vi "find_handle_pose_update.vi"(8 "Manipulator pose":T7 format="%#_5f", 9 "Light 3":sgl[](array[numeric]), 10 "Parameters":T1={"Stimulus"={"Type"=enum."Off", "Delay"=0, "Amplitude"=[0.0, 0.0, 0.0], "Injection point"=enum."Total pose", "Closed loop"=FALSE, "Offset"=[0.0, 0.0, 0.0], "Tip -> world"=TRUE}, "Goal Filter A"={"Lower Fc"=0.0, "Lower Q"=0.15, "Scale factor"=0.0, "Upper Fc"=0.0075, "Upper Q"=0.01, "Manip zeroing"=0.001, "Speedup max"=150.0, "Speedup thresh"=5.0, "Speedup nonlin"=3.0, "V limit"=300.0, "V limit range"=300.0}, "Mode controls"={"Hold"=FALSE, "Cancellation"=FALSE, "Goal filter"=FALSE, "Trigger"=FALSE}, "Manipulator type"=enum."Current piezo", "Manipulator calibration"={"Inverse Kinematics"=[[-0.4736411481566654, -0.25724305819165183, -1.1087933259307599], [0.296735958809338, -0.258643951607561, -1.0971603505753995], [-0.043664688535758014, 0.44635679599468125, -1.1035515399424176]], "Handle transform"=[[3.281333089700394, 0.23462731743748497, 0.17832137948371765, -8265.081657965618], [-0.20249098046098263, 2.6933210343964133, -0.2815002765708058, -33565.66155248382], [-0.14581170473284072, 0.6821648518522063, 0.8833544952169589, 26862.18782130476], [-1.1202010727438122e-18, 5.861467994999758e-19, 1.760134464394436e-18, 0.999999999999992]], "Tip offset"=[0.0, 0.0, 36200.0], "Probe calibration"=[], "Pivot position"=[0.0, 0.0, -11360.0], "Axial filter"={"filter structure"=enum."IIR 2nd Order", "Reverse Coefficients"=[0.0, 0.0], "Forward Coefficients"=[1.0, 0.0, 0.0]}, "Lateral filter"={"filter structure"=enum."IIR 2nd Order", "Reverse Coefficients"=[0.0, 0.0], "Forward Coefficients"=[1.0, 0.0, 0.0]}}, "Charge piezo"={"Capacitance"=4e-08, "V min"=-235.0, "V max"=50.0, "- margin"=465.0, "+ margin"=0.001, "I max"=40000.0, "I sat"=90000000.0, "R series"=5.0, "R shunt"=1000.0, "Fault V"=0.0, "Start Fault V"=0.0, "Start Cycles"=0, "Prop gain"=1e-06, "Int gain"=0.0, "Diff gain"=0.0}, "Network"={"Remote Host"="192.168.1.3", "Send Status"=TRUE, "Send Port"=0, "Recv Commands"=FALSE, "Recv Port"=0}, "Goal Filter B"={"Lower Fc"=1.0, "Lower Q"=2.0, "Scale factor"=61557.0, "Upper Fc"=20.0, "Upper Q"=61557.0, "Manip zeroing"=2.0, "Speedup max"=1.0, "Speedup thresh"=300.0, "Speedup nonlin"=3.0, "V limit"=300.0, "V limit range"=300.0}, "Cancellation"={"Bandwidth"=0.0, "Delay"=0, "Stack travel"=0.0, "Saturation pos"=0.0075, "Slew Limit"=0.01, "Turnoff zeroing"=0.001, "Bypass"=FALSE}, "Transition time"=3.0} {"Transition time" format="%_3f"; "Cancellation"."Slew Limit" format="%#_3p"; "Cancellation"."Saturation pos" format="%#.1f"; "Cancellation"."Stack travel" format="%#.1f"; "Cancellation"."Turnoff zeroing" format="%#_6e"; "Cancellation"."Delay" step=1; "Cancellation"."Bandwidth" min=10 max=1000 step=10; "Goal Filter B"."V limit range" format="%_3p"; "Goal Filter B"."V limit" format="%_3p"; "Goal Filter B"."Speedup nonlin" format="%_3p"; "Goal Filter B"."Upper Q" format="%_3f"; "Goal Filter B"."Upper Fc" format="%_3p"; "Goal Filter B"."Lower Q" format="%_3f"; "Goal Filter B"."Speedup thresh" format="%_3p"; "Goal Filter B"."Speedup max" format="%_3p"; "Goal Filter B"."Manip zeroing" format="%_3p"; "Goal Filter B"."Scale factor" format="%_3f"; "Goal Filter B"."Lower Fc" format="%_3p"; "Charge piezo"."I sat" format="%#_6p"; "Charge piezo"."+ margin" format="%#_6p"; "Charge piezo"."- margin" format="%#_6p"; "Charge piezo"."Start Fault V" format="%#_6p"; "Charge piezo"."R shunt" format="%#_6p"; "Charge piezo"."Prop gain" format="%#_6p"; "Charge piezo"."Fault V" format="%#_6p"; "Charge piezo"."I max" format="%#_6p"; "Charge piezo"."Diff gain" format="%#_6p"; "Charge piezo"."Int gain" format="%#_6p"; "Charge piezo"."R series" format="%#_6p"; "Charge piezo"."Capacitance" format="%#_6p"; "Manipulator calibration"."Probe calibration" format="%#.1f"; "Manipulator calibration"."Handle transform" format="%#_3f"; "Manipulator calibration"."Inverse Kinematics" format="%#_3f"; "Goal Filter A"."V limit range" format="%_3p"; "Goal Filter A"."V limit" format="%_3p"; "Goal Filter A"."Speedup nonlin" format="%_3p"; "Goal Filter A"."Upper Q" format="%_3f"; "Goal Filter A"."Upper Fc" format="%_3p"; "Goal Filter A"."Lower Q" format="%_3f"; "Goal Filter A"."Speedup thresh" format="%_3p"; "Goal Filter A"."Speedup max" format="%_3p"; "Goal Filter A"."Manip zeroing" format="%_3p"; "Goal Filter A"."Scale factor" format="%_3f"; "Goal Filter A"."Lower Fc" format="%_3p"; "Stimulus"."Offset" step=100; "Stimulus"."Amplitude" step=100; "Stimulus"."Delay" step=100}) -> (0 "Central tip position":sgl[](array[numeric]), 1 "Tip position":sgl[](array[numeric]), 2 "Handle Rotation":T7 format="%#_5f", 3 "Handle Translation":sgl[](array[numeric]))   [LabVIEW 2010]
uses:
  <vilib>/Analysis/Matrix/Datatypes/RealMatrix.ctl
  testing/Micron params.ctl
  testing/stimulus.ctl
  testing/injection_point.ctl
  filtering/goal_filter_parms.ctl
  testing/mode_conrols.ctl
  testing/manipulator_cal.ctl
  asap/labview/testing/probe_calibration.ctl
  manipulator/Charge controller params.ctl
  host/network_params.ctl
  cancellation/im_control_params.ctl
  <vilib>/Analysis/baseanly.llb/A x Vector.vi
  utilities/labview/norm_vec.vi
  <vilib>/Analysis/NI_AALBase.lvlib
  <vilib>/Analysis/Matrix/NI_Matrix.lvlib
panel:
  # "Offset to apply to central tip position to keep manipulator centered."
  # "Tip position in world coordinates"
  # "Manipulator pose as computed in in the main micron_update loop and stored in the \"Manipulator pose\" shared var."
  # "Intended tip position implied by handle pose."
  # "Pose of the handle.  When the tip is centered, the handle and manipulator pose are identical."
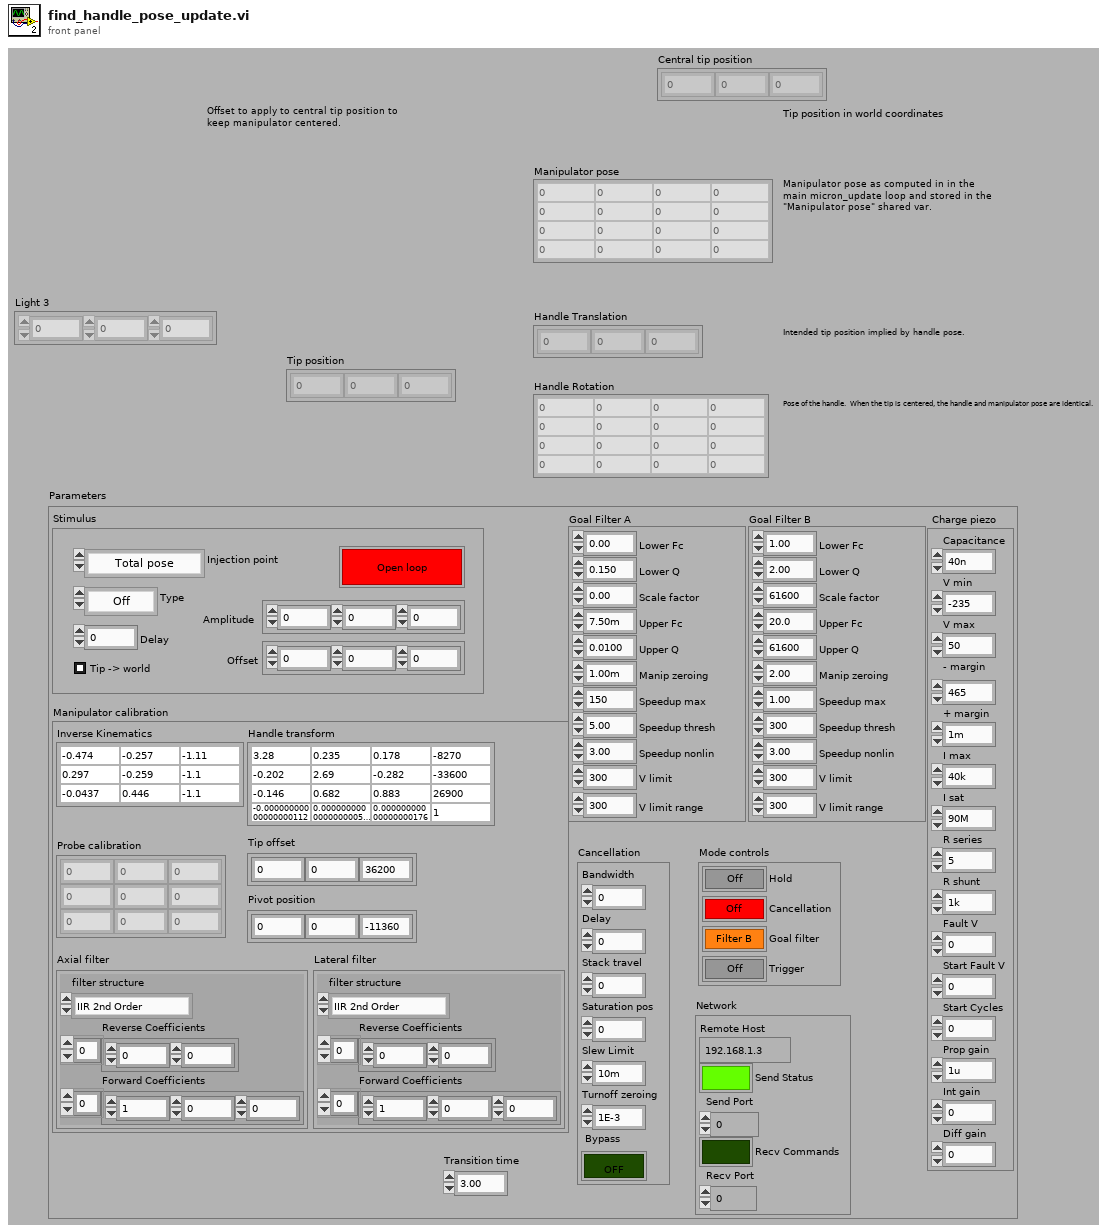
[diagram p1: front panel]
types:
  T1 = typedef "Micron params.ctl" = cluster{"Stimulus":T2, "Goal Filter A":T4, "Mode controls":T5, "Manipulator type":enum16{"Current piezo", "Voltage piezo"}, "Manipulator calibration":T6, "Charge piezo":T9, "Network":T10, "Goal Filter B":T4, "Cancellation":T11, "Transition time":sgl}
  T2 = typedef "stimulus.ctl" = cluster{"Type":enum16{"Off", "Step", "Sine", "Triangle", "Arbitrary"}, "Delay":i32, "Amplitude":sgl[], "Injection point":T3, "Closed loop":bool, "Offset":sgl[], "Tip -> world":bool}
  T3 = typedef "injection_point.ctl" = enum16{"Total pose", "V limiter", "Goal position", "Tip error (manip)", "Inverse kin", "Controller", "Stack position", "Stack drive", "DAC"}
  T4 = typedef "goal_filter_parms.ctl" = cluster{"Lower Fc":sgl, "Lower Q":sgl, "Scale factor":sgl, "Upper Fc":sgl, "Upper Q":sgl, "Manip zeroing":sgl, "Speedup max":sgl, "Speedup thresh":sgl, "Speedup nonlin":sgl, "V limit":sgl, "V limit range":sgl}
  T5 = typedef "mode_conrols.ctl" = cluster{"Hold":bool, "Cancellation":bool, "Goal filter":bool, "Trigger":bool}
  T6 = typedef "manipulator_cal.ctl" = cluster{"Inverse Kinematics":T7, "Handle transform":T7, "Tip offset":sgl[], "Probe calibration":T8, "Pivot position":sgl[], "Axial filter":cluster{"filter structure":enum32{"IIR 2nd Order", "IIR 4th Order"}, "Reverse Coefficients":dbl[], "Forward Coefficients":dbl[]}, "Lateral filter":cluster{"filter structure":enum32{"IIR 2nd Order", "IIR 4th Order"}, "Reverse Coefficients":dbl[], "Forward Coefficients":dbl[]}}
  T7 = typedef "NI_Matrix.lvlib/RealMatrix.ctl" = dbl[][]
  T8 = typedef "probe_calibration.ctl" = sgl[][]
  T9 = typedef "Charge controller params.ctl" = cluster{"Capacitance":sgl, "V min":sgl, "V max":sgl, "- margin":sgl, "+ margin":sgl, "I max":sgl, "I sat":sgl, "R series":sgl, "R shunt":sgl, "Fault V":sgl, "Start Fault V":sgl, "Start Cycles":i32, "Prop gain":sgl, "Int gain":sgl, "Diff gain":sgl}
  T10 = typedef "network_params.ctl" = cluster{"Remote Host":string, "Send Status":bool, "Send Port":u16, "Recv Commands":bool, "Recv Port":u16}
  T11 = typedef "im_control_params.ctl" = cluster{"Bandwidth":sgl, "Delay":i32, "Stack travel":sgl, "Saturation pos":sgl, "Slew Limit":sgl, "Turnoff zeroing":sgl, "Bypass":bool}
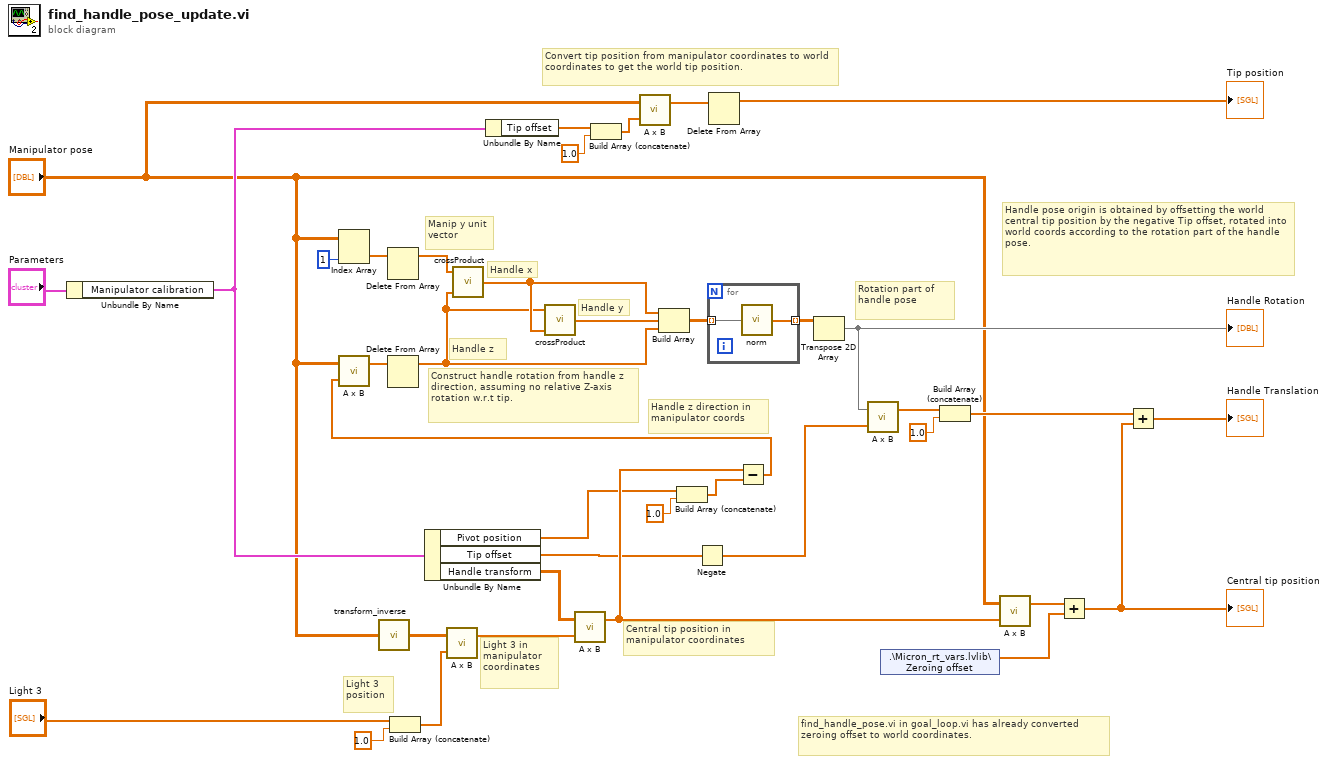
[diagram p0: block diagram]
diagram:
  # "Convert tip position from manipulator coordinates to world coordinates to get the world tip position."
  # "Handle pose origin is obtained by offsetting the world central tip position by the negative Tip offset, rotated into world coords according to the rotation part of the handle pose."
  # "find_handle_pose.vi in goal_loop.vi has already converted zeroing offset to world coordinates."
  # "Rotation part of handle pose"
  # "Handle z direction in manipulator coords"
  # "Central tip position in manipulator coordinates"
  # "Light 3 in manipulator  coordinates"
  # "Light 3 position"
  # "Construct handle rotation from handle z direction, assuming no relative Z-axis rotation w.r.t tip."
  # "Handle y"
  # "Handle x"
  # "Handle z"
  # "Manip y unit vector"
  n1 = Unbundle By Name("Parameters") -> ("Manipulator calibration"=w4:T6)
  n2 = Index Array(array="Manipulator pose", index (col)=1 ("disabled index (col)")) -> (element=w38:dbl[])  [unwired: 1 in]
  n3 = call "transform_inverse.vi"("Transform"="Manipulator pose") -> ("Inverse transform"=w29:T7)
  n4 = Delete From Array(array=w38) -> (array with subset deleted=w35:dbl[])  [unwired: 2 in, 1 out]
  n5 = Build Array (concatenate)("Light 3", sgl 1.0) -> (w27:sgl[])
  n6 = Unbundle By Name(w4) -> ("Pivot position"=w21:sgl[], "Tip offset"=w16:sgl[], "Handle transform"=w20:T7)
  n7 = call-poly <vilib>:"A x B.vi"("Vector"=w27, "A"=w29) -> ("A x Vector"=w26:dbl[])  [unwired: 1 out]
  n8 = Unbundle By Name(w4) -> ("Tip offset"=w5:sgl[])
  n9 = call-poly <vilib>:"A x B.vi"("Vector"=w26, "A"=w20) -> ("A x Vector"=w24:dbl[])  [unwired: 1 out]
  n10 = Build Array (concatenate)(w5, sgl 1.0 ("Numeric")) -> (w6:sgl[])
  n11 = call-poly <vilib>:"A x B.vi"("Vector"=w6, "A"="Manipulator pose") -> ("A x Vector"=w7:dbl[])  [unwired: 1 out]
  n12 = Build Array (concatenate)(w21, sgl 1.0 ("Numeric")) -> (w19:sgl[])
  n13 = Negate(x=w16) -> (-x=w15:sgl[])
  n14 = Delete From Array(array=w7) -> (array with subset deleted=→"Tip position":dbl[])  [unwired: 2 in, 1 out]
  n15 = Subtract(x=w24, y=w19) -> (x-y=w25:dbl[])
  n16 = call-poly <vilib>:"A x B.vi"("Vector"=w25, "A"="Manipulator pose") -> ("A x Vector"=w36:dbl[])  [unwired: 1 out]
  n17 = Delete From Array(array=w36) -> (array with subset deleted=w32:dbl[])  [unwired: 2 in, 1 out]
  n18 = call "crossProduct.vi"("B"=w32, "A"=w35) -> ("A x B"=w34:dbl[])  [unwired: 3 out]
  n19 = call "crossProduct.vi"("B"=w34, "A"=w32) -> ("A x B"=w33:dbl[])  [unwired: 3 out]
  n20 = Build Array(w34, w33, w32) -> (w31:dbl[][])
  n21 = for {
    tunnel: w31 -> [w40] mode=indexing
    tunnel: [w39] -> w30 mode=indexing
    n22 = call-poly "norm.vi"("vector"=w40) -> ("normalized vector"=w39:dbl[])  [unwired: 4 out]
  }
  n23 = Transpose 2D Array(2D array=w30) -> (transposed array=w9:dbl[][])
  "Handle Rotation" <- w9
  n24 = call-poly <vilib>:"A x B.vi"("Vector"=w15, "A"=w9) -> ("A x Vector"=w13:dbl[])  [unwired: 1 out]
  n25 = shared-variable ".\\Micron_rt_vars.lvlib\\Zeroing offset"() -> (w17:sgl[])  [unwired: 2 out]
  n26 = Build Array (concatenate)(w13, sgl 1.0 ("Numeric")) -> (w12:dbl[])
  n27 = call-poly <vilib>:"A x B.vi"("Vector"=w24, "A"="Manipulator pose") -> ("A x Vector"=w18:dbl[])  [unwired: 1 out]
  n28 = Add(x=w18, y=w17) -> (x+y=w2:dbl[])
  "Central tip position" <- w2
  n29 = Add(x=w12, y=w2) -> (x+y=→"Handle Translation":dbl[])
